vi "Read Offset.vi"(8 "error in (no error)":errorcluster, 11 "CAN_RW_CORE in":refnum<class "L2ENET_RW_CORE.lvclass">) -> (0 "error out":errorcluster, 2 "Offset":i32, 3 "CAN_RW_CORE out":refnum<class "L2ENET_RW_CORE.lvclass">)   [LabVIEW 2021, in "L2ENET_RW_CORE.lvclass"]
uses:
  L2ENET_RW_CORE.lvclass
  L2ENET_RW_CORE.lvclass/L2ENET_RW_CORE.ctl
  <vilib>/CIF Foundation/CIF PCAP Parse and Build/pcap_Parse_Build_CIF.lvclass/pcap_Parse_Build_CIF.ctl
  <vilib>/CIF Foundation/CIF PCAP Parse and Build/pcap_Parse_Build_CIF.lvclass
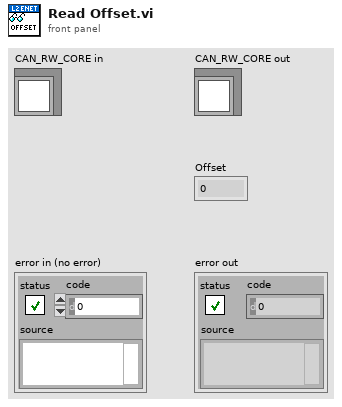
[diagram p1: front panel]
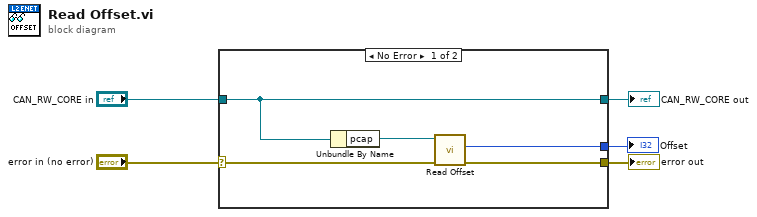
[diagram p0: block diagram]
diagram:
  n1 = case shown="No Error" "error in (no error)" {
    selector: "error in (no error)" -> [w8 w11]
    tunnel: [w7 w11] -> w4
    tunnel: [w10 w12] -> w2
    tunnel: "CAN_RW_CORE in" -> [w10 w12]
    tunnel: [w6 _] -> w1
    frame No Error {
      n2 = Unbundle By Name(w10) -> ("pcap"=w9:refnum<class "pcap_Parse_Build_CIF.lvclass">)
      n3 = call <vilib>:"Read Offset.vi"("error in (no error)"=w8, "pcap Parse and Build in"=w9) -> ("error out"=w7:errorcluster, "Offset"=w6:i32)  [unwired: 7 in, 1 out]
    }
    frame Error {
    }
  }
  "error out" <- w4
  "CAN_RW_CORE out" <- w2
  "Offset" <- w1
